vi "Close.vi"(8 "error in":errorcluster, 11 "writer":refnum<class "Synnax Writer.lvclass">) -> (0 "error out":errorcluster)   [LabVIEW 2026, in "synnax_clib.lvlib" / "Synnax Writer.lvclass"]
doc: "SYNNAX_EXPORT int32_t synnax_writer_close(SynnaxWriter writer, SynnaxError err);"
uses:
  Synnax Writer.lvclass
  Synnax Writer.lvclass/Synnax Writer.ctl
  synnax_clib.dll
  synnax_clib.lvlib
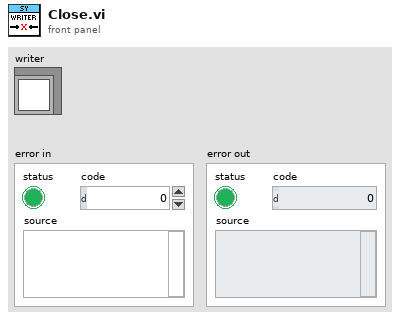
[diagram p1: front panel]
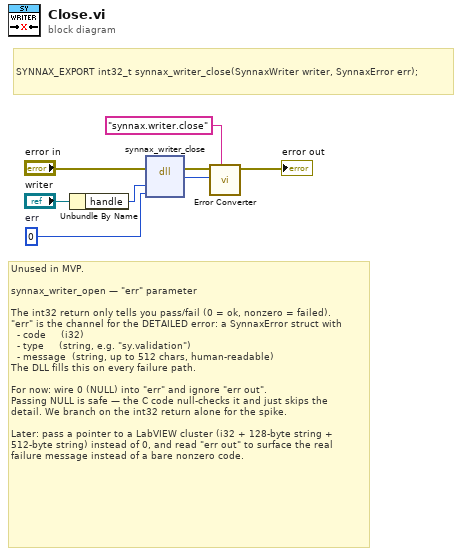
[diagram p0: block diagram]
diagram:
  w8 = u64 0  # err
  # "Unused in MVP.\n\nsynnax_writer_open — \"err\" parameter\n\nThe int32 return only tells you pass/fail (0 = ok, nonzero = failed).\n\"err\" is the channel for the DETAILED error: a SynnaxError struct with\n  - code     (i32)\n  - type     (string, e.g. \"sy.validation\")\n  - message  (string, up to 512 chars, human-readable)\nThe DLL fills this on every failure path.\n\nFor now: wire 0 (NULL) into \"err\" and ignore \"err out\".\nPassing NULL is safe — the C code null-checks it and just skips the\ndetail. We branch on the int32 return alone for the spike.\n\nLater: pass a pointer to a LabVIEW cluster (i32 + 128-byte string +\n512-byte string) instead of 0, and read \"err out\" to surface the real\nfailure message instead of a bare nonzero code."
  # "SYNNAX_EXPORT int32_t synnax_writer_close(SynnaxWriter writer, SynnaxError err);"
  n1 = Unbundle By Name("writer") -> ("handle"=w1:u64)
  n2 = dll-call lib="C/synnax/client/labview/synnax_clib.*" fn="synnax_writer_close"(error in="error in", "writer"=w1, "err"=w8) -> (error out=w7:errorcluster, w6:i32)  [unwired: 4 in, 1 out]
  n3 = call "Error Converter.vi"("source"="synnax.writer.close", "error code"=w6, "error in (no error)"=w7) -> ("error out"=→"error out":errorcluster)  [unwired: 8 in]
